vi "Main.vi"() -> ()   [LabVIEW 2013]
uses:
  <vilib>/ULx/Create Channel.llb/ULx Create Channel (AI-Voltage-Basic).vi
  <vilib>/ULx/Timing.llb/ULx Timing (Sample Clock).vi
  <vilib>/ULx/Read.llb/ULx Read (Analog Wfm 1Chan 1Samp).vi
  <vilib>/ULx/Create Channel.llb/ULx Create Channel (CI-Frequency).vi
  <vilib>/ULx/Read.llb/ULx Read (Counter DBL 1Chan 1Samp).vi
panel:
  in  "sample mode 2":i32(ring) items=["FiniteSamples", "ContinuousSamples"]
  in  "samples per channel 2":i32=1000
  in  "clock source 2":i32(ring) items=["OnboardClock", "ExternalClock", "NoClock"]
  in  "rate 2":dbl=1000.0
  in  "error in 2":errorcluster
  in  "physical channels 2":refnum<k21>
  in  "stop 3":bool
  out "Numeric 2":i32
  out "Waveform Chart 3":waveform(dbl)(graph)
  in  "stop 2":bool
  out "Waveform Chart 2":dbl(graph)
  in  "counters":refnum<k21>
  out "Numeric":i32
  out "Waveform Chart":waveform(dbl)(graph)
  in  "sample mode":i32(ring) items=["FiniteSamples", "ContinuousSamples"]
  in  "samples per channel":i32=1000
  in  "clock source":i32(ring) items=["OnboardClock", "ExternalClock", "NoClock"]
  in  "rate":dbl=1000.0
  in  "error in":errorcluster
  in  "physical channels":refnum<k21>
  in  "stop":bool
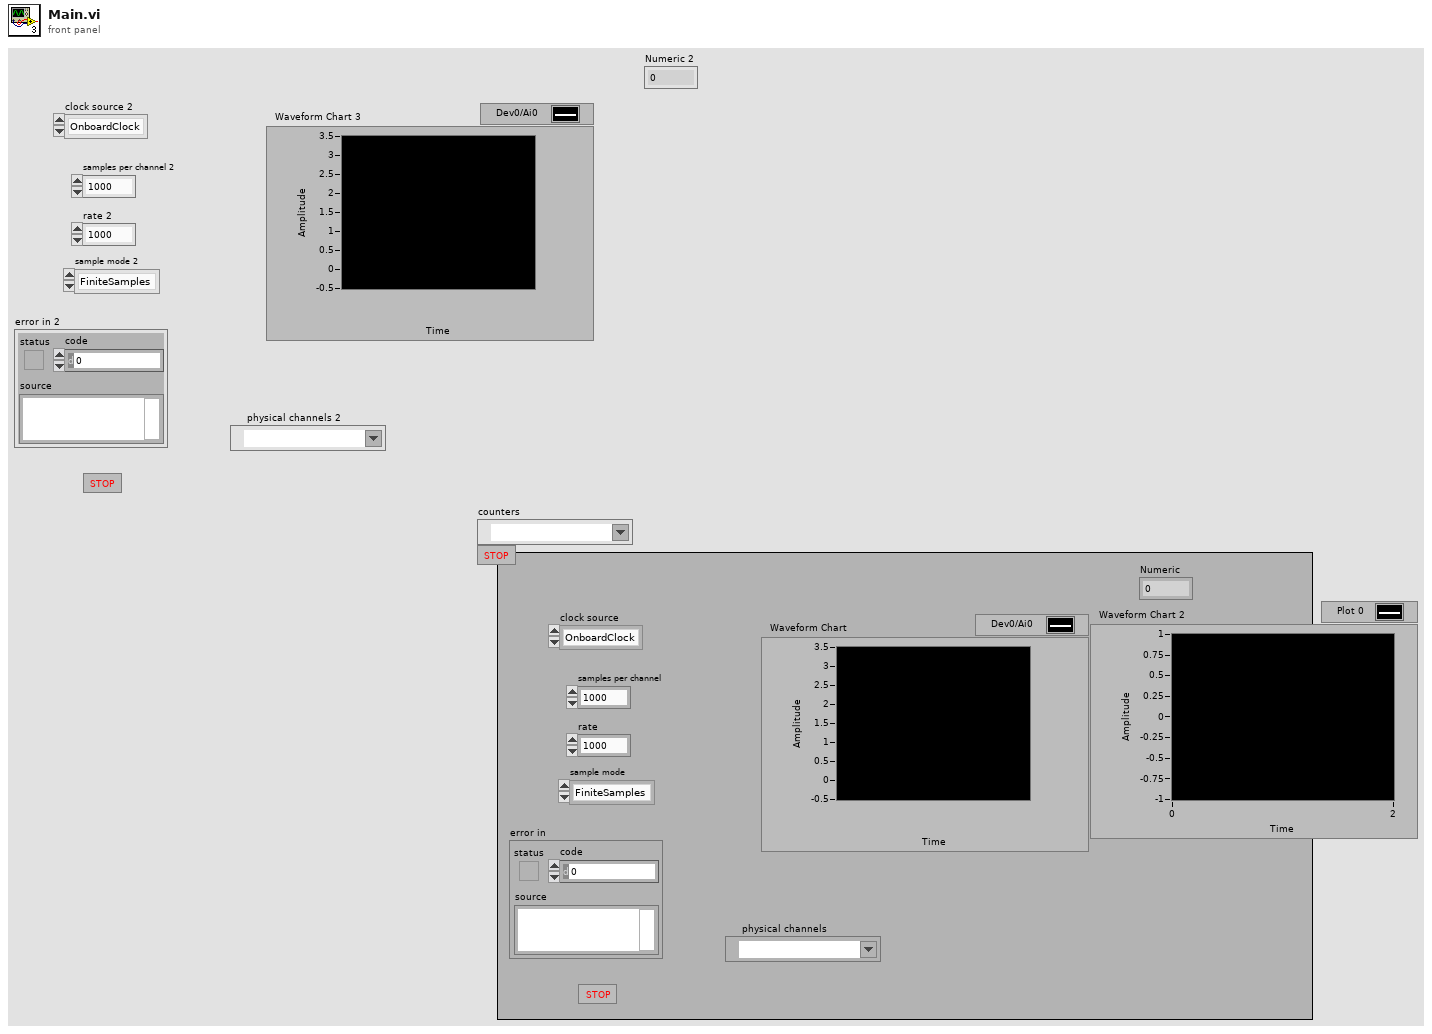
[diagram p1: front panel]
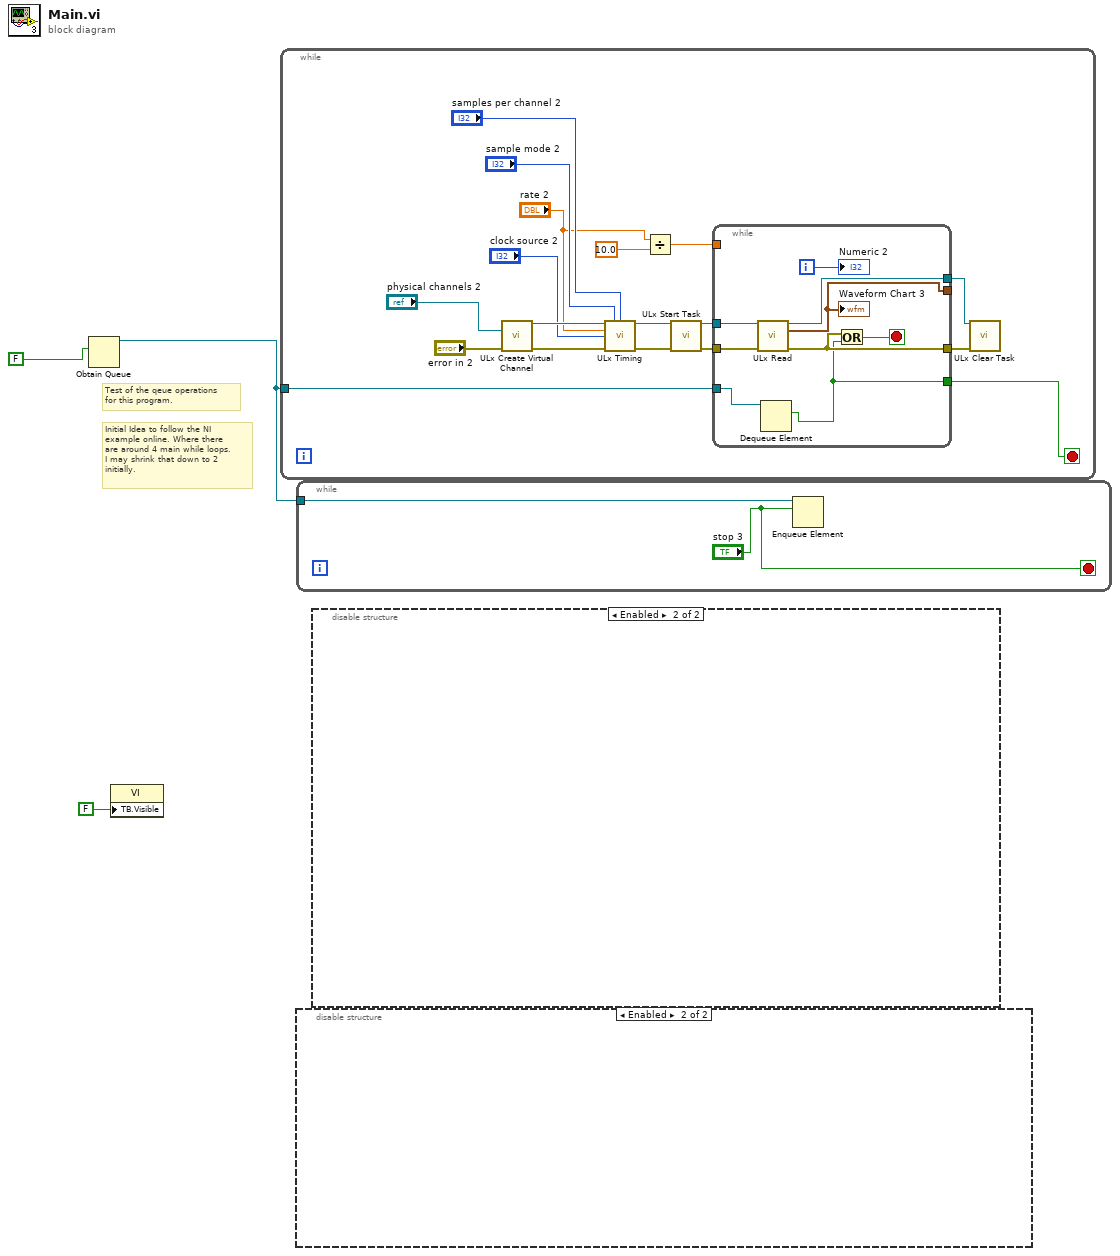
[diagram p0: block diagram]
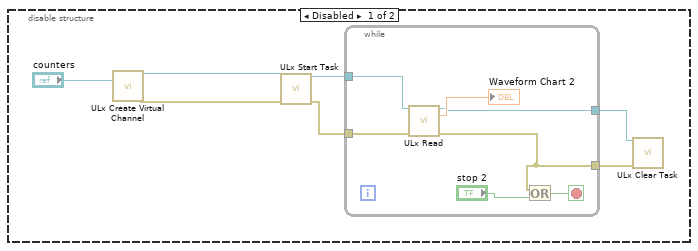
[diagram p2: hidden frame]
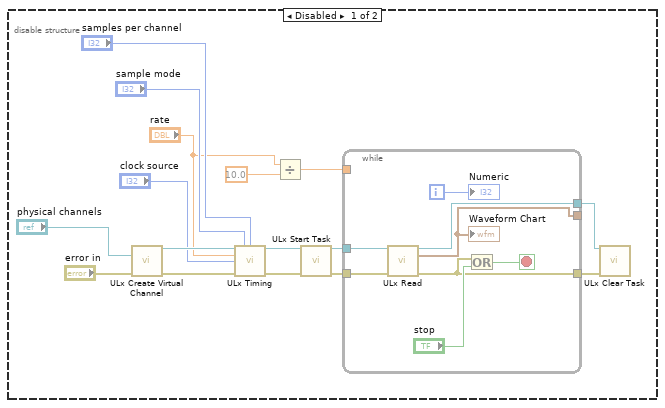
[diagram p3: hidden frame]
diagram:
  # "Initial Idea to follow the NI\nexample online. Where there\nare around 4 main while loops.\nI may shrink that down to 2\ninitially."
  # "Test of the qeue operations\nfor this program."
  n1 = Obtain Queue(element data type=FALSE ("stop 3")) -> (queue out=w1:refnum<queue>)  [unwired: 4 in, 2 out]
  n2 = property class="VI"("TB.Visible"=FALSE ("Tool Bar:Visible")) -> ()  [unwired: 2 in, 2 out]
  n3 = while {
    tunnel: w1 -> [w5]
    stop <- w4 stop-if-true
    n4 = call-poly <vilib>:"ULx Create Virtual Channel.vi"("physical channels"="physical channels 2", "error in"="error in 2") -> ("task out"=w19:refnum<k24>, "error out"=w18:errorcluster)  [unwired: 12 in]
    n5 = call-poly <vilib>:"ULx Timing.vi"("task in"=w19, "sample mode"="sample mode 2", "samples per channel"="samples per channel 2", "rate"="rate 2", "clock source"="clock source 2", "error in"=w18) -> ("task out"=w14:refnum<k24>, "error out"=w13:errorcluster)  [unwired: 8 in]
    n6 = Divide(x="rate 2", y=10.0) -> (x/y=w6:dbl)
    n7 = call <vilib>:"ULx Start Task.vi"("task in"=w14, "error in"=w13) -> ("task out"=w12:refnum<k24>, "error out"=w11:errorcluster)  [unwired: 12 in]
    n8 = while {
      tunnel: w12 -> [w30]
      tunnel: w11 -> [w29]
      tunnel: [w27] -> w10
      tunnel: [w25] -> w9
      tunnel: [w24] -> _
      tunnel: w6 -> [_]
      tunnel: w5 -> [w23]
      tunnel: [w22] -> w4
      i -> [w28]
      stop <- w26 stop-if-true
      n9 = call-poly <vilib>:"ULx Read.vi"("task in"=w30, "error in"=w29) -> ("task out"=w27:refnum<k24>, "data"=w24:waveform(dbl), "error out"=w25:errorcluster)  [unwired: 11 in]
      "Waveform Chart 3" <- w24
      n10 = Dequeue Element(queue=w23) -> (element=w22:bool)  [unwired: 2 in, 3 out]
      n11 = Or(x=w25, y=w22) -> (x .or. y?=w26:bool)
      "Numeric 2" <- w28
    }
    n12 = call <vilib>:"ULx Clear Task.vi"("task in"=w10, "error in"=w9) -> ()  [unwired: 13 in, 1 out]
  }
  n13 = while {
    tunnel: w1 -> [w32]
    stop <- "stop 3" stop-if-true
    n14 = Enqueue Element(queue=w32, element="stop 3") -> ()  [unwired: 2 in, 3 out]
  }
  n15 = disable-structure shown="Enabled" {
    frame Disabled {
      n16 = call-poly <vilib>:"ULx Create Virtual Channel.vi"("counters"="counters") -> ("task out"=w35:refnum<k24>, "error out"=w36:errorcluster)  [unwired: 13 in]
      n17 = call <vilib>:"ULx Start Task.vi"("task in"=w35, "error in"=w36) -> ("task out"=w38:refnum<k24>, "error out"=w37:errorcluster)  [unwired: 12 in]
      n18 = while {
        tunnel: w38 -> [w45]
        tunnel: w37 -> [w44]
        tunnel: [w41] -> w34
        tunnel: [w43] -> w33
        stop <- w42 stop-if-true
        n19 = call-poly <vilib>:"ULx Read.vi"("task in"=w45, "error in"=w44) -> ("task out"=w43:refnum<k24>, "data"=→"Waveform Chart 2":dbl, "error out"=w41:errorcluster)  [unwired: 11 in]
        n20 = Or(x=w41, y="stop 2") -> (x .or. y?=w42:bool)
      }
      n21 = call <vilib>:"ULx Clear Task.vi"("task in"=w33, "error in"=w34) -> ()  [unwired: 13 in, 1 out]
    }
    frame Enabled {
    }
  }
  n22 = disable-structure shown="Enabled" {
    frame Disabled {
      n23 = call-poly <vilib>:"ULx Create Virtual Channel.vi"("physical channels"="physical channels", "error in"="error in") -> ("task out"=w60:refnum<k24>, "error out"=w59:errorcluster)  [unwired: 12 in]
      n24 = call-poly <vilib>:"ULx Timing.vi"("task in"=w60, "sample mode"="sample mode", "samples per channel"="samples per channel", "rate"="rate", "clock source"="clock source", "error in"=w59) -> ("task out"=w55:refnum<k24>, "error out"=w54:errorcluster)  [unwired: 8 in]
      n25 = Divide(x="rate", y=10.0) -> (x/y=w47:dbl)
      n26 = call <vilib>:"ULx Start Task.vi"("task in"=w55, "error in"=w54) -> ("task out"=w53:refnum<k24>, "error out"=w52:errorcluster)  [unwired: 12 in]
      n27 = while {
        tunnel: w53 -> [w70]
        tunnel: w52 -> [w69]
        tunnel: [w67] -> w51
        tunnel: [w64] -> w50
        tunnel: [w63] -> _
        tunnel: w47 -> [_]
        i -> [w68]
        stop <- w65 stop-if-true
        n28 = call-poly <vilib>:"ULx Read.vi"("task in"=w70, "error in"=w69) -> ("task out"=w67:refnum<k24>, "data"=w63:waveform(dbl), "error out"=w64:errorcluster)  [unwired: 11 in]
        "Waveform Chart" <- w63
        n29 = Or(x=w64, y="stop") -> (x .or. y?=w65:bool)
        "Numeric" <- w68
      }
      n30 = call <vilib>:"ULx Clear Task.vi"("task in"=w51, "error in"=w50) -> ()  [unwired: 13 in, 1 out]
    }
    frame Enabled {
    }
  }
